vi "Borders and Shading Constant (Table) Shell.vi"   [LabVIEW 2010]
doc: "Defines the borders and shading attributes of a table in Word."
uses:
  <vilib>/addons/_office/NI_ReportGenerationToolkit.lvlib
types:
  T1 = cluster{"OutsideLineStyle":i32, "OutsideColor":i32, "OutsideLineWidth":i32, "InsideLineStyle":i32, "InsideColor":i32, "InsideLineWidth":i32, "BackgroundPatternColor":i32}
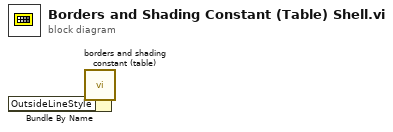
[diagram p0: block diagram]
diagram:
  n1 = call <vilib>:"borders and shading constant (table).vi"() -> ("borders and shading"=w1:T1)
  n2 = Bundle By Name(cluster=w1) -> ()  [unwired: 1 in, 1 out]
